vi "Test INI Settings.vi"(11 "Test Case In":refnum<class "INI Settings.lvclass">) -> (0 "error out":errorcluster, 3 "Test Case Out":refnum<class "INI Settings.lvclass">)   [LabVIEW 2021, in "INI Settings.lvclass"]
uses:
  INI Settings.lvclass
  C:/Program Files/National Instruments/LabVIEW 2025/vi.lib/Astemes/LUnit/Test Case.lvclass
  <vilib>/Astemes/LUnit/Test Case.lvclass/Test Case.ctl
  INI Settings.lvclass/INI Settings.ctl
  4993e8ee-a06a-463a-9684-69129f64d5ce.vi
  <vilib>/LabVIEW Icon API/lv_icon/lv_icon.lvlib
  <vilib>/LabVIEW Icon API/lv_icon/Controls/Font.ctl
  <vilib>/LabVIEW Icon API/lv_icon/Controls/Alignment.ctl
  <resource>/plugins/NIIconEditor/Controls/Font Size.ctl
  <vilib>/LabVIEW Icon API/lv_icon/Controls/BodyText.ctl
  <vilib>/LabVIEW Icon API/lv_icon/Controls/IEColor.ctl
  <resource>/plugins/NIIconEditor/Controls/Tools.ctl
  <resource>/plugins/NIIconEditor/INI/INI Data.ctl
panel:
  in  "Font ComboBox":string(combo)
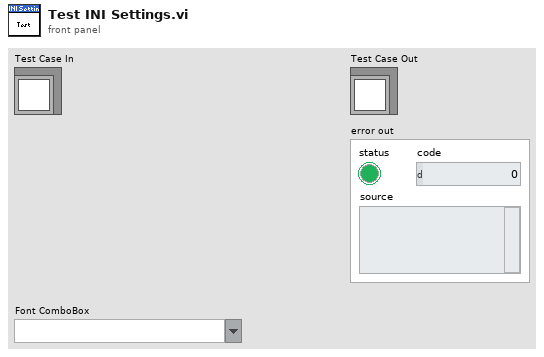
[diagram p1: front panel]
types:
  T1 = typedef "lv_icon.lvlib/INI Data.ctl" = cluster{"Show Terminals?":bool, "Text":cluster{"Font":T2, "Alignment":T3, "Size":T4}, "3rd party Templates":cluster{"Store 3rd party Templates?":bool, "Folder Name":string}, "Merge user layers on commit":bool, "Body Text":T5, "Fill Color":T6, "Edge Color":T6, "Tab":u16, "Tool":T7, "Disable Layers?":bool}
  T2 = typedef "Font.ctl" = string
  T3 = typedef "Alignment.ctl" = u16
  T4 = typedef "Font Size.ctl" = u8
  T5 = typedef "BodyText.ctl" = cluster{"Line 1 text":string, "Line 2 text":string, "Line 3 text":string, "Line 4 text":string, "Line 1 color":u32, "Line 2 color":u32, "Line 3 color":u32, "Line 4 color":u32, "Body Text Spec":cluster{"Font":T2, "Alignment":T3, "Size":u8}, "Center text vertically":bool, "Capitalize Text":bool}
  T6 = typedef "IEColor.ctl" = u32
  T7 = typedef "Tools.ctl" = enum32{"Pencil", "Line", "Dropper", "Fill", "Rectangle", "Filled Rectangle", "Ellipse", "Filled Ellipse", "Eraser", "Text", "Select", "Move"}
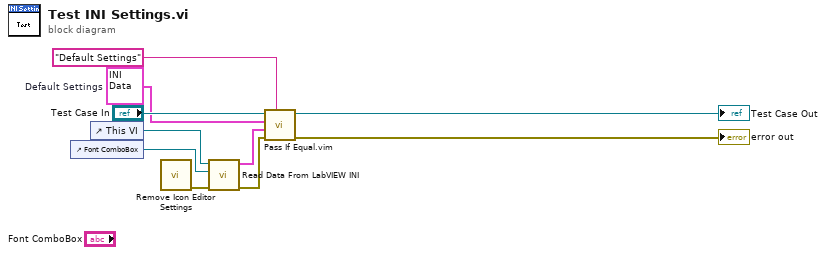
[diagram p0: block diagram]
diagram:
  w2 = T1 {"Show Terminals?"=FALSE, "Text"={"Font"="Small Fonts", "Alignment"=1, "Size"=9}, "3rd party Templates"={"Store 3rd party Templates?"=TRUE, "Folder Name"="3rd party"}, "Merge user layers on commit"=FALSE, "Body Text"={"Line 1 text"="", "Line 2 text"="", "Line 3 text"="", "Line 4 text"="", "Line 1 color"=0, "Line 2 color"=0, "Line 3 color"=0, "Line 4 color"=0, "Body Text Spec"={"Font"="Small Fonts", "Alignment"=1, "Size"=9}, "Center text vertically"=TRUE, "Capitalize Text"=TRUE}, "Fill Color"=16711680, "Edge Color"=0, "Tab"=0, "Tool"=enum."Pencil", "Disable Layers?"=FALSE}  # Default Settings
  n1 = control-ref of="Font ComboBox"() -> (w4:refnum<vi>)
  n2 = control-ref of="This VI"() -> (w5:refnum<vi>)
  n3 = call "Remove Icon Editor Settings.vi"() -> ("error out"=w9:errorcluster)  [unwired: 11 in]
  n4 = call <resource>:"Read Data From LabVIEW INI.vi"("error in"=w9, "DNL_Font"=w4, "IE VI Ref"=w5) -> ("error out"=w8:errorcluster, "INI Data"=w1:T1)  [unwired: 7 in]
  n5 = call "Pass If Equal.vim"("Description"="Default Settings", "error in (no error)"=w8, "Actual"=w1, "Expected"=w2, "LUnit Test Case In"="Test Case In") -> ("error out"=→"error out":errorcluster, "LUnit Test Case Out"=→"Test Case Out":refnum<class "INI Settings.lvclass">)  [unwired: 5 in]
